vi "Intialise VL Patch image frames.vi"(8 "error in (no error)":errorcluster, 11 "Experiment Parameters":T2) -> (0 "error out":errorcluster, 3 "VL Image Refs":T1[](array[typedef]))   [LabVIEW 2020]
uses:
  Typedefs/Experiment Parameters.ctl
  <vilib>/vision/Image Controls.llb/IMAQ Image.ctl
  Timelapse Viewer/Globals/gl_Time series viewer globals.vi
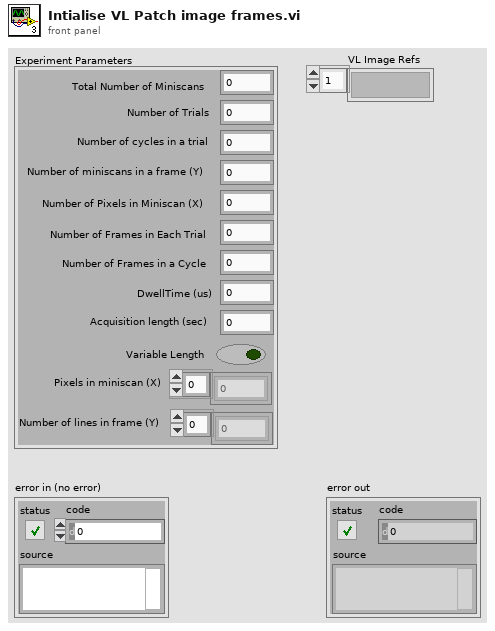
[diagram p1: front panel]
types:
  T1 = typedef "IMAQ Image.ctl" = refnum<image>
  T2 = typedef "Experiment Parameters.ctl" = cluster{"Total Number of Miniscans":i32, "Number of Trials":i32, "Number of cycles in a trial":i32, "Number of miniscans in a frame (Y)":i32, "Number of Pixels in Miniscan (X)":i32, "Number of Frames in Each Trial":i32, "Number of Frames in a Cycle":i32, "DwellTime (us)":dbl, "Acquisition length (sec)":dbl, "Variable Length":bool, "Pixels in miniscan (X)":dbl[], "Number of lines in frame (Y)":dbl[]}
  T3 = typedef "Time series viewer refs.ctl" = cluster{"This VI":refnum<vi>, "Image control":refnum<vi>, "AVI Mode ind":refnum<vi>, "Play":refnum<vi>, "Stop":refnum<vi>, "Back":refnum<vi>, "Scrollbar":refnum<vi>, "Video length info":refnum<vi>, "Expected speed values":refnum<vi>, "Intensity":refnum<vi>, "Path":refnum<vi>, "Selection sliders":refnum<vi>, "Speed Graph ref":refnum<vi>, "Frame rate set (fps)":refnum<vi>, "Number of rows to generate":refnum<vi>, "VL Image Array":refnum<vi>, "Image Scrollbar":refnum<vi>, "Channel to load":refnum<vi>, "Colour":refnum<vi>}
  T4 = typedef "Channel to load.ctl" = enum16{"Show red channel", "Show green channel", "Show both channels"}
  T5 = typedef "Image Type" = u32
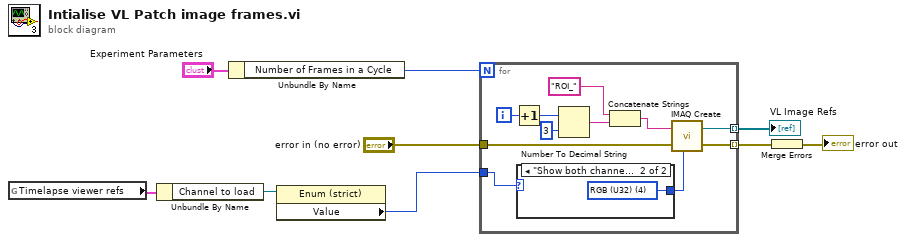
[diagram p0: block diagram]
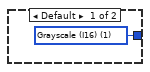
[diagram p2: hidden frame]
diagram:
  n1 = global read "gl_Time series viewer globals.vi" "Timelapse viewer refs"() -> (w3:T3)
  n2 = Unbundle By Name(w3) -> ("Channel to load"=w2:refnum<vi>)
  n3 = Unbundle By Name("Experiment Parameters") -> ("Number of Frames in a Cycle"=w8:i32)
  n4 = property class="Enum (strict)"(reference=w2) -> ("Value"=w1:T4)  [unwired: 1 in, 2 out]
  n5 = for {
    N: w8 -> [_]
    tunnel: "error in (no error)" -> [w13]
    tunnel: [w12] -> w6 mode=indexing
    tunnel: [w11] -> w4 mode=indexing
    tunnel: w1 -> [w10]
    i -> [w19]
    n6 = Increment(x=w19) -> (x+1=w18:i32)
    n7 = case shown="\"Show both channels\"" w10 {
      tunnel: [w21 w22] -> w20
      frame Default {
        w21 = T5 1 items=["Grayscale (U8)", "Grayscale (I16)", "Grayscale (SGL)", "Complex (CSG)", "RGB (U32)", "HSL (U32)", "RGB (U64)", "Grayscale (U16)"] ("Image Type")
      }
      frame "Show both channels" {
        w22 = T5 4 items=["Grayscale (U8)", "Grayscale (I16)", "Grayscale (SGL)", "Complex (CSG)", "RGB (U32)", "HSL (U32)", "RGB (U64)", "Grayscale (U16)"] ("Image Type")
      }
    }
    n8 = Number To Decimal String(number=w18, width (-)=i16 3) -> (decimal integer string=w15:string)
    n9 = Concatenate Strings("ROI_" ("Image Name"), w15) -> (w14:string)
    n10 = call "IMAQ Create"("Image Name"=w14, "Image Type"=w20, "error in (no error)"=w13) -> ("New Image"=w11:T1, "error out"=w12:errorcluster)  [unwired: 1 in, 1 out]
  }
  "VL Image Refs" <- w4
  n11 = Merge Errors(w6) -> (→"error out":errorcluster)
